vi "ProperMoveChecker.vi"(10 "Possible Squares":i32[][](array[numeric]), 11 "Clicked Square":i32[](array[numeric])) -> (3 "Enable?":bool)   [LabVIEW 2019]
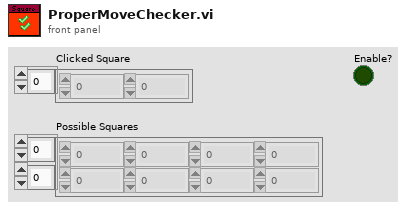
[diagram p1: front panel]
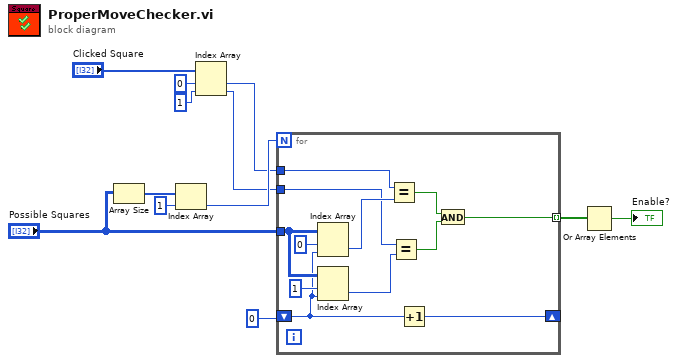
[diagram p0: block diagram]
diagram:
  n1 = Array Size(array="Possible Squares") -> (size(s)=w9:i32[])
  n2 = Index Array(array=w9, index=1) -> (element=w11:i32)
  n3 = Index Array(array="Clicked Square", index #1=0 ("index"), index #2=1 ("index")) -> (element #1=w3:i32, element #2=w4:i32)
  n4 = for {
    N: w11 -> [_]
    tunnel: "Possible Squares" -> [w21]
    tunnel: w3 -> [w19]
    tunnel: w4 -> [w17]
    shift-right: [w24] -> _
    shift-left: 0 ("index") -> [w20]
    tunnel: [w13] -> w6 mode=indexing
    n5 = Index Array(array=w21, index (row)=0, index (col)=w20) -> (element=w18:i32)
    n6 = Index Array(array=w21, index (row)=1, index (col)=w20) -> (element=w16:i32)
    n7 = Equal?(x=w19, y=w18) -> (x = y?=w15:bool)
    n8 = Equal?(x=w17, y=w16) -> (x = y?=w14:bool)
    n9 = Increment(x=w20) -> (x+1=w24:i32)
    n10 = And(x=w15, y=w14) -> (x .and. y?=w13:bool)
  }
  n11 = Or Array Elements(Boolean array=w6) -> (logical OR=→"Enable?":bool)
